vi "Read_Flow_Press_Bkgd.vi"() -> ()   [LabVIEW 2016]
uses:
  <vilib>/Analysis/baseanly.llb/Mean (DBL).vi
  <userlib>/Fluigent/Fluigent MFCS/FluigentMFCS_Full.llb/MFCS_EZ Detect.vi
  <userlib>/Fluigent/Fluigent MFCS/FluigentMFCS_Full.llb/MFCS_EZ Initialization.vi
  <userlib>/Fluigent/Fluigent MFCS/FluigentMFCS_Full.llb/MFCS_EZ Read All Channels Pressure.vi
  <userlib>/Fluigent/Fluigent MFCS/FluigentMFCS_Full.llb/MFCS_EZ Close.vi
  <vilib>/Analysis/NI_AALBase.lvlib
panel:
  in  "Flow 2 Filter Size":dbl
  out "freq (Hz) 2":dbl
  out "Sample Rate":dbl(graph)
  in  "Values to Display":dbl=100.0
  out "Flow Rates":T1(graph)
  in  "milliseconds to wait":u32
  in  "stop 2":bool
  out "dP/dt":dbl(graph)
  in  "reset":bool
  out "Histogram Graph":T2(graph)
  in  "Flow 1 Filter Size":dbl
  out "freq (Hz)":dbl
  in  "stop":bool
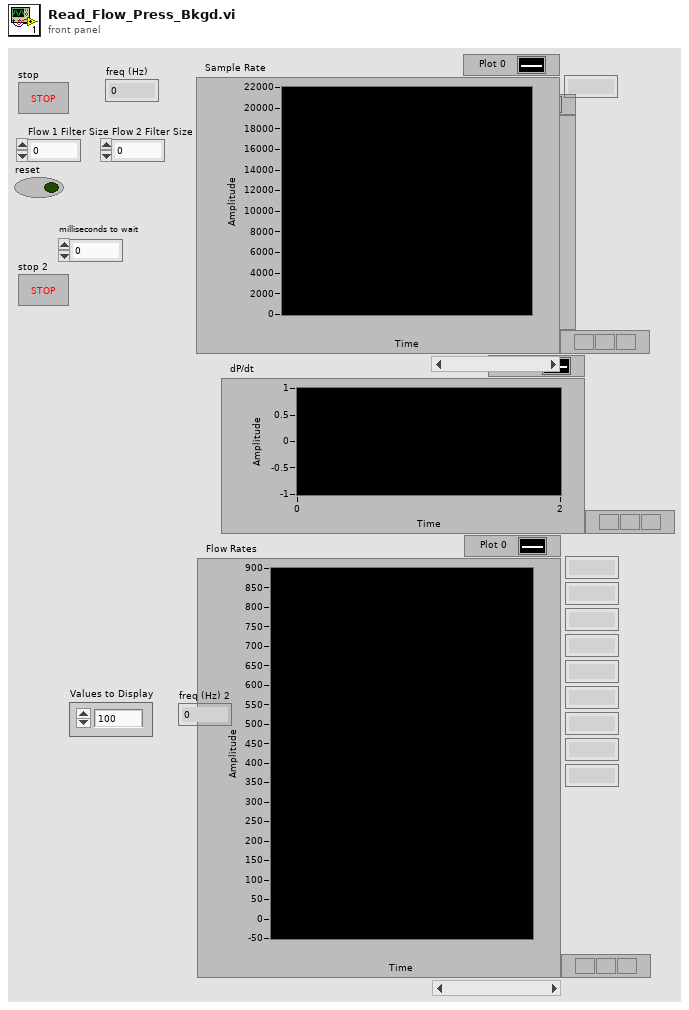
[diagram p1: front panel]
types:
  T1 = cluster{"[0]":dbl, "[1]":dbl, "[2]":dbl, "[3]":dbl, "[4]":dbl, "[5]":dbl, "[6]":dbl, "[7]":dbl, "[8]":dbl}
  T2 = cluster{"X Values":dbl[], "Histogram: h(x)":i32[]}
  T3 = typedef "_EZmfcsSN.ctl" = u16
  T4 = typedef "_frpRefNum" = refnum<k1>
  T5 = typedef "_EZmfcsRefNum.ctl" = refnum<k1>
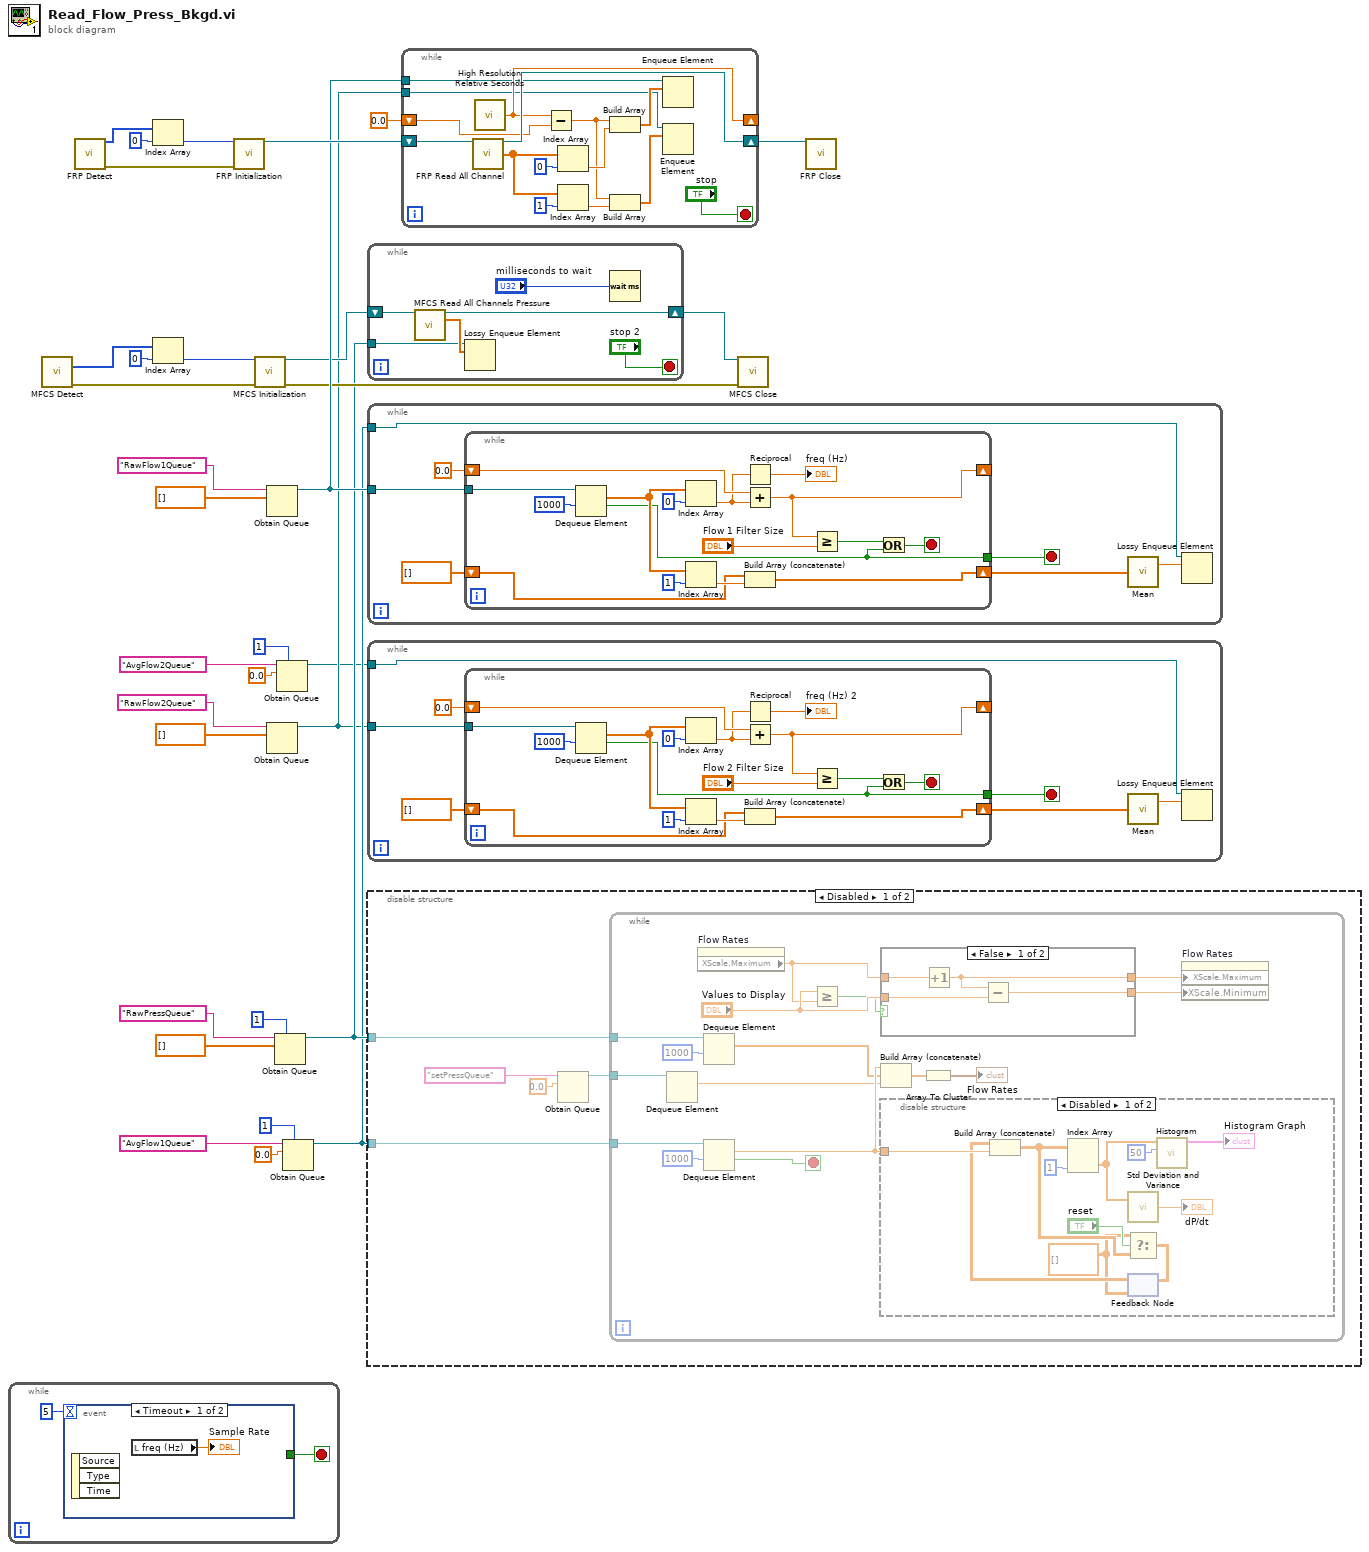
[diagram p0: block diagram]
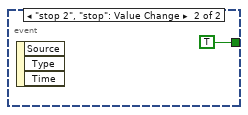
[diagram p2: hidden frame]
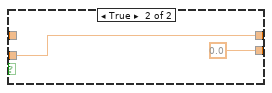
[diagram p3: hidden frame]
diagram:
  n1 = while {
    stop <- w33 stop-if-true
    n2 = event shown="[0] Timeout" {
      selector: _ -> [_ _]
      dyn-events: _ -> [_ _]
      timeout: 5 -> [_ _]
      tunnel: [_ TRUE] -> w33
      event Timeout {
        n3 = event-data() -> ()  [unwired: 1 in, 3 out]
        n4 = local read "freq (Hz)"() -> (→"Sample Rate":dbl)
      }
      event "stop 2", "stop": Value Change {
        n5 = event-data() -> ()  [unwired: 1 in, 3 out]
      }
    }
  }
  n6 = call-poly <userlib>:"MFCS Detect.vi"() -> ("[SN MFCS_EZ]"=w22:T3[], "error out"=w20:errorcluster)  [unwired: 14 in]
  n7 = call <userlib>:"FRP Detect.vi"() -> ("FLOWBOARD List"=w32:u16[], "error out"=w30:errorcluster)  [unwired: 14 in]
  n8 = Index Array(array=w32, index=0) -> (element=w29:u16)
  n9 = Index Array(array=w22, index=0) -> (element=w21:T3)
  n10 = call <userlib>:"FRP Initialization.vi"("Serial Number"=w29, "error in (no error)"=w30) -> ("FRP out"=w28:T4)  [unwired: 11 in, 2 out]
  n11 = call-poly <userlib>:"MFCS Initialization.vi"("SN MFCS_EZ"=w21, "error in (no error)"=w20) -> ("MFCS_EZ"=w18:T5, "error out"=w16:errorcluster)  [unwired: 11 in, 1 out]
  n12 = Obtain Queue(name (unnamed)="RawFlow1Queue", element data type=dbl[] [] ("appended array")) -> (queue out=w25:refnum<queue>)  [unwired: 3 in, 2 out]
  n13 = Obtain Queue(name (unnamed)="RawFlow2Queue", element data type=dbl[] [] ("appended array")) -> (queue out=w6:refnum<queue>)  [unwired: 3 in, 2 out]
  n14 = Obtain Queue(max queue size (-1, unlimited)=1, name (unnamed)="RawPressQueue", element data type=dbl[] [] ("appended array")) -> (queue out=w10:refnum<queue>)  [unwired: 2 in, 2 out]
  n15 = Obtain Queue(max queue size (-1, unlimited)=1, name (unnamed)="AvgFlow2Queue", element data type=0.0 ("mean")) -> (queue out=w3:refnum<queue>)  [unwired: 2 in, 2 out]
  n16 = Obtain Queue(max queue size (-1, unlimited)=1, name (unnamed)="AvgFlow1Queue", element data type=0.0 ("mean")) -> (queue out=w9:refnum<queue>)  [unwired: 2 in, 2 out]
  n17 = while {
    shift-right: [w40] -> w17
    shift-left: w18 -> [w41]
    tunnel: w10 -> [w37]
    stop <- "stop 2" stop-if-true
    n18 = call-poly <userlib>:"MFCS Read All Channels Pressure.vi"("MFCS_EZ"=w41) -> ("MFCS_EZ out"=w40:T5, "All Channels Pressure"=w39:dbl[])  [unwired: 12 in, 1 out]
    n19 = Lossy Enqueue Element(queue=w37, element=w39) -> ()  [unwired: 1 in, 4 out]
    n20 = Wait (ms)(milliseconds to wait="milliseconds to wait") -> ()  [unwired: 1 out]
  }
  n21 = while {
    tunnel: w25 -> [w49]
    tunnel: w9 -> [w46]
    stop <- w47 stop-if-true
    n22 = while {
      tunnel: w49 -> [w65]
      shift-right: [w54] -> _
      shift-left: 0.0 ("Flow-Rate") -> [w63]
      tunnel: [w55] -> w47
      shift-right: [w51] -> w44
      shift-left: dbl[] [] -> [w50]
      stop <- w56 stop-if-true
      n23 = Dequeue Element(queue=w65, timeout in ms (-1)=1000) -> (element=w61:dbl[], timed out?=w55:bool)  [unwired: 1 in, 2 out]
      n24 = Index Array(array=w61, index=0) -> (element=w52:dbl)
      n25 = Index Array(array=w61, index=1) -> (element=w59:dbl)
      n26 = Reciprocal(x=w52) -> (1/x=→"freq (Hz)":dbl)
      n27 = Add(x=w63, y=w52) -> (x+y=w54:dbl)
      n28 = Build Array (concatenate)(w50, w59) -> (w51:dbl[])
      n29 = Greater Or Equal?(x=w54, y="Flow 1 Filter Size") -> (x >= y?=w57:bool)
      n30 = Or(x=w57, y=w55) -> (x .or. y?=w56:bool)
    }
    n31 = call-poly <vilib>:"Mean.vi"("X"=w44) -> ("mean"=w43:dbl)  [unwired: 1 out]
    n32 = Lossy Enqueue Element(queue=w46, element=w43) -> ()  [unwired: 1 in, 4 out]
  }
  n33 = while {
    tunnel: w6 -> [w72]
    tunnel: w3 -> [w69]
    stop <- w70 stop-if-true
    n34 = while {
      tunnel: w72 -> [w88]
      shift-right: [w77] -> _
      shift-left: 0.0 ("Flow-Rate") -> [w86]
      tunnel: [w78] -> w70
      shift-right: [w74] -> w67
      shift-left: dbl[] [] -> [w73]
      stop <- w79 stop-if-true
      n35 = Dequeue Element(queue=w88, timeout in ms (-1)=1000) -> (element=w84:dbl[], timed out?=w78:bool)  [unwired: 1 in, 2 out]
      n36 = Index Array(array=w84, index=0) -> (element=w75:dbl)
      n37 = Index Array(array=w84, index=1) -> (element=w82:dbl)
      n38 = Reciprocal(x=w75) -> (1/x=→"freq (Hz) 2":dbl)
      n39 = Add(x=w86, y=w75) -> (x+y=w77:dbl)
      n40 = Build Array (concatenate)(w73, w82) -> (w74:dbl[])
      n41 = Greater Or Equal?(x=w77, y="Flow 2 Filter Size") -> (x >= y?=w80:bool)
      n42 = Or(x=w80, y=w78) -> (x .or. y?=w79:bool)
    }
    n43 = call-poly <vilib>:"Mean.vi"("X"=w67) -> ("mean"=w66:dbl)  [unwired: 1 out]
    n44 = Lossy Enqueue Element(queue=w69, element=w66) -> ()  [unwired: 1 in, 4 out]
  }
  n45 = disable-structure shown="Disabled" {
    disable-tunnel: w9 -> [w93 _]
    disable-tunnel: w10 -> [w92 _]
    frame Disabled {
      n46 = Obtain Queue(name (unnamed)="setPressQueue", element data type=0.0) -> (queue out=w89:refnum<queue>)  [unwired: 3 in, 2 out]
      n47 = while {
        tunnel: w93 -> [w108]
        tunnel: w92 -> [w106]
        tunnel: w89 -> [w95]
        stop <- w105 stop-if-true
        n48 = Dequeue Element(queue=w95) -> (element=w94:dbl)  [unwired: 2 in, 3 out]
        n49 = property on="Flow Rates" class="WFChart (strict)"() -> ("XScale.Maximum"=w98:dbl)  [unwired: 2 in, 2 out]
        n50 = Dequeue Element(queue=w106, timeout in ms (-1)=1000) -> (element=w103:dbl[])  [unwired: 1 in, 3 out]
        n51 = Dequeue Element(queue=w108, timeout in ms (-1)=1000) -> (element=w104:dbl, timed out?=w105:bool)  [unwired: 1 in, 2 out]
        n52 = Greater Or Equal?(x="Values to Display", y=w98) -> (x >= y?=w99:bool)
        n53 = case shown="False" w99 {
          tunnel: "Values to Display" -> [w111 w115]
          tunnel: w98 -> [w113 _]
          tunnel: [w110 w115] -> w96
          tunnel: [w112 0.0] -> w97
          frame False {
            n54 = Increment(x=w113) -> (x+1=w110:dbl)
            n55 = Subtract(x=w110, y=w111) -> (x-y=w112:dbl)
          }
          frame True {
          }
        }
        n56 = Build Array (concatenate)(w104, w103, w94) -> (w101:dbl[])
        n57 = disable-structure shown="Disabled" {
          disable-tunnel: w104 -> [w126 _]
          frame Disabled {
            w119 = dbl[][] []
            n58 = feedback #1(w119) -> (w125:dbl[][])
            n59 = Build Array (concatenate)(w125, w126) -> (w120:dbl[][])
            n60 = Index Array(array=w120, index (col)=1 ("disabled index (col)")) -> (element=w117:dbl[])  [unwired: 1 in]
            n61 = call <vilib>:"Std Deviation and Variance.vi"("X"=w117) -> ("standard deviation"=→"dP/dt":dbl)  [unwired: 1 in, 2 out]
            n62 = Select(t=w119, s="reset", f=w120) -> (s? t:f=w118:dbl[][])
            n63 = feedback-in #1(w118) -> ()
            n64 = call <vilib>:"Histogram.vi"("intervals"=50, "X"=w117) -> ("Histogram Graph"=→"Histogram Graph":T2)  [unwired: 6 in, 3 out]
          }
          frame Enabled {
          }
        }
        n65 = Array To Cluster(array=w101) -> (cluster=→"Flow Rates":T1)
        n66 = property on="Flow Rates" class="WFChart (strict)"("XScale.Maximum"=w96, "XScale.Minimum"=w97) -> ()  [unwired: 2 in, 2 out]
      }
    }
    frame Enabled {
    }
  }
  n67 = while {
    shift-right: [w140] -> w27
    shift-left: w28 -> [w141]
    shift-right: [w137] -> _
    shift-left: 0.0 ("relative seconds") -> [w138]
    tunnel: w25 -> [w135]
    tunnel: w6 -> [w127]
    stop <- "stop" stop-if-true
    n68 = call <userlib>:"FRP Read All Channel.vi"("FRP"=w141) -> ("FRP out"=w140:T4, "All Flow-Rates"=w131:dbl[])  [unwired: 12 in, 1 out]
    n69 = call <vilib>:"High Resolution Relative Seconds.vi"() -> ("relative seconds"=w137:dbl)
    n70 = Subtract(x=w137, y=w138) -> (x-y=w130:dbl)
    n71 = Index Array(array=w131, index=0) -> (element=w133:dbl)
    n72 = Index Array(array=w131, index=1) -> (element=w129:dbl)
    n73 = Build Array(w130, w133) -> (w136:dbl[])
    n74 = Build Array(w130, w129) -> (w128:dbl[])
    n75 = Enqueue Element(queue=w135, element=w136) -> ()  [unwired: 2 in, 3 out]
    n76 = Enqueue Element(queue=w127, element=w128) -> ()  [unwired: 2 in, 3 out]
  }
  n77 = call-poly <userlib>:"MFCS Close.vi"("MFCS_EZ"=w17, "error in (no error)"=w16) -> ()  [unwired: 13 in, 1 out]
  n78 = call <userlib>:"FRP Close.vi"("FRP"=w27) -> ()  [unwired: 14 in, 1 out]
